vi "GOOPUtil_CompareRootClass.vi"(0 "GOOP Object 1":refnum<class>, 1 "GOOP Object 2":refnum<class>, 5 "error in (no error)":errorcluster) -> (14 "SameAncestor":bool, 15 "GOOPObject1Ancestors":string[](array[string]), 16 "GOOPObject2Ancestors":string[](array[string]), 19 "error out":errorcluster)   [LabVIEW 2012, in "GOOPUtility.lvlib"]
doc: "Compares the two GOOP object references and checks if they have the same ancestor type.\n\nThis is a collection of generic GOOP utility VIs. Please notice that it is important that the frontpanel of the Create, Destroy and GetObjectStatus is not removed when building an application."
uses:
  <vilib>/addons/GOOPUtility/GOOPUtility.lvlib
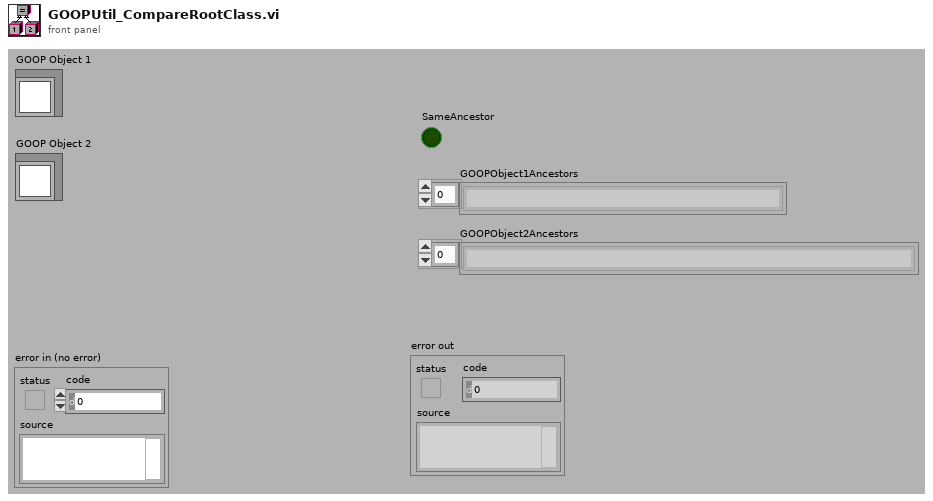
[diagram p1: front panel]
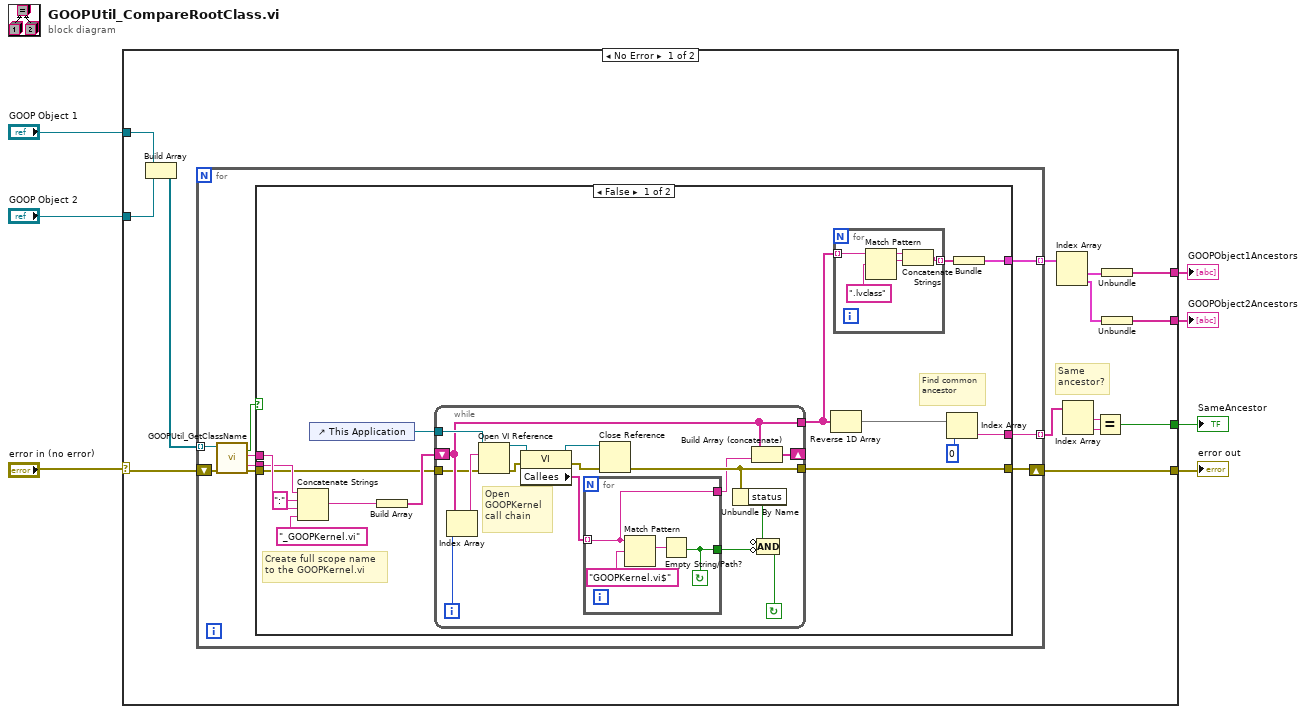
[diagram p0: block diagram]
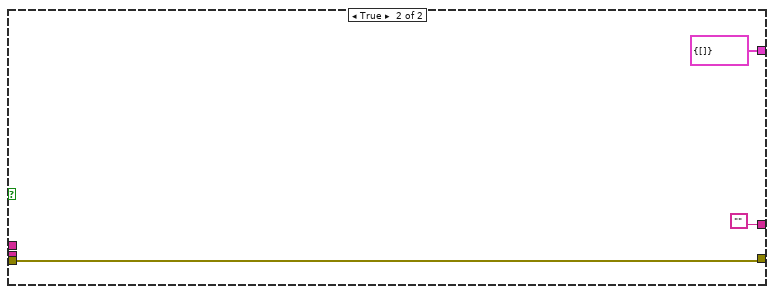
[diagram p2: hidden frame]
diagram:
  n1 = case shown="No Error" "error in (no error)" {
    selector: "error in (no error)" -> [w21 w74]
    tunnel: "GOOP Object 1" -> [w20 _]
    tunnel: "GOOP Object 2" -> [w19 _]
    tunnel: [w17 w74] -> w4
    tunnel: [w13 _] -> w3
    tunnel: [w9 _] -> w2
    tunnel: [w8 _] -> w1
    frame No Error {
      # "Same\nancestor?"
      n2 = Build Array(w20, w19) -> (w18:refnum<class>[])
      n3 = for {
        shift-right: [w24] -> w17
        shift-left: w21 -> [w25]
        tunnel: w18 -> [w23] mode=indexing
        tunnel: [w28] -> w16 mode=indexing
        tunnel: [w27] -> w12 mode=indexing
        n4 = call <vilib>:"GOOPUtil_GetClassName.vi"("LabVIEW Object"=w23, "error in (no error)"=w25) -> ("IsEmptyObject?"=w22:bool, "Class Name"=w30:string, "Full Class Name"=w29:string, "error out"=w26:errorcluster)  [unwired: 13 in, 1 out]
        n5 = case shown="False" w22 {
          tunnel: w30 -> [w45 _]
          tunnel: w29 -> [w42 _]
          tunnel: [w36 ""] -> w28
          tunnel: [w35 cluster{string[]} {[]}] -> w27
          tunnel: w26 -> [w32 w73]
          tunnel: [w31 w73] -> w24
          frame False {
            # "Find common\nancestor"
            # "Create full scope name\nto the GOOPKernel.vi"
            n6 = Concatenate Strings(w42, ":" ("string"), w45, "_GOOPKernel.vi" ("name or relative path")) -> (w40:string)
            n7 = control-ref of="This Application"() -> (w43:refnum<vi>)
            n8 = Build Array(w40) -> (w39:string[])
            n9 = while {
              tunnel: w43 -> [w65]
              tunnel: [w56] -> w31
              shift-right: [w54] -> _
              shift-left: w39 -> [w53]
              tunnel: [w53] -> w34
              tunnel: w32 -> [w51]
              i -> [w59]
              stop <- w57 continue-if-true
              # "Open\nGOOPKernel\ncall chain"
              n10 = Index Array(array=w53, index=w59) -> (element=w60:string)
              n11 = Open VI Reference(application reference (local)=w65, vi path=w60, error in (no error)=w51) -> (vi reference=w63:refnum<vi>, error out=w64:errorcluster)  [unwired: 3 in]
              n12 = property class="VI"(reference=w63, error in=w64) -> (reference out=w62:refnum<vi>, error out=w66:errorcluster, "Callees"=w61:string[])
              n13 = for {
                tunnel: w61 -> [w67] mode=indexing
                tunnel: [w68] -> w58
                tunnel: [w67] -> w52
                stop <- w68 continue-if-true
                n14 = Match Pattern(string=w67, regular expression="GOOPKernel.vi$") -> (match substring=w69:string)  [unwired: 1 in, 3 out]
                n15 = Empty String/Path?(string/path=w69) -> (empty?=w68:bool)
              }
              n16 = Close Reference(reference=w62, error in (no error)=w66) -> (error out=w56:errorcluster)
              n17 = Unbundle By Name(w56) -> ("status"=w55:bool)
              n18 = Build Array (concatenate)(w53, w52) -> (w54:string[])
              n19 = Compound Arithmetic op=AND(invert w55, invert w58) -> (w57:bool)
            }
            n20 = Reverse 1D Array(array=w34) -> (reversed array=w38:string[])
            n21 = for {
              tunnel: w34 -> [w47] mode=indexing
              tunnel: [w46] -> w33 mode=indexing
              n22 = Match Pattern(string=w47, regular expression=".lvclass") -> (before substring=w49:string, match substring=w48:string)  [unwired: 1 in, 2 out]
              n23 = Concatenate Strings(w49, w48) -> (w46:string)
            }
            n24 = Index Array(array=w38, index=0) -> (element=w36:string)
            n25 = Bundle(w33) -> (w35:cluster{string[]})  [unwired: 1 in]
          }
          frame True {
          }
        }
      }
      n26 = Index Array(array=w12) -> (element #1=w11:cluster{string[]}, element #2=w10:cluster{string[]})  [unwired: 2 in]
      n27 = Index Array(array=w16) -> (element #1=w15:string, element #2=w14:string)  [unwired: 2 in]
      n28 = Equal?(x=w15, y=w14) -> (x = y?=w13:bool)
      n29 = Unbundle(w11) -> (w9:string[])
      n30 = Unbundle(w10) -> (w8:string[])
    }
    frame Error {
    }
  }
  "error out" <- w4
  "SameAncestor" <- w3
  "GOOPObject1Ancestors" <- w2
  "GOOPObject2Ancestors" <- w1
